vi "GetMethodDependency.vi"(0 "ClassReaderNative in":refnum<class "ClassReaderNative.lvclass">, 1 "Method(s)":variant, 5 "error in (no error)":errorcluster) -> (14 "ClassReaderNative out":refnum<class "ClassReaderNative.lvclass">, 15 "DependencyVIs":T1[](array[typedef]), 19 "error out":errorcluster)   [LabVIEW 2012, in "ClassReaderNative.lvclass"]
uses:
  <resource>/Framework/Providers/Open_GDS/ClassProviders/Provider_LvNativeClass/ClassReaderNative_class/ClassReaderNative.lvclass
  <resource>/Framework/Providers/Open_GDS/ClassProviders/Provider_BaseClassInterface/ClassReader_class/MethodDependencyType.ctl
  <resource>/Framework/Providers/Open_GDS/ClassProviders/Common/ScriptingFunctions/SubVIs/Scripting_ViDependencyType.ctl
  <resource>/Framework/Providers/Open_GDS/ClassProviders/Provider_BaseClassInterface/ClassReader_class/ClassReader.lvclass
  <resource>/Framework/Providers/Open_GDS/ClassProviders/Provider_LvNativeClass/ClassReaderNative_class/ClassReaderNative.lvclass/ClassReaderNative.ctl
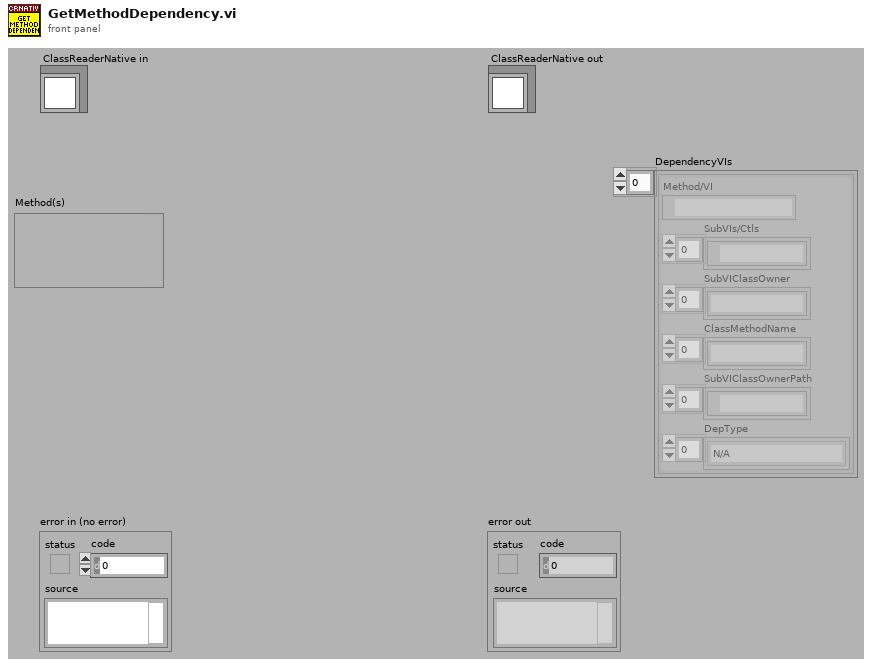
[diagram p1: front panel]
types:
  T1 = typedef "MethodDependencyType.ctl" = cluster{"Method/VI":path, "SubVIs/Ctls":path[], "SubVIClassOwner":string[], "ClassMethodName":string[], "SubVIClassOwnerPath":path[], "DepType":T2[]}
  T2 = typedef "Scripting_ViDependencyType.ctl" = enum16{"N/A", "Launches"}
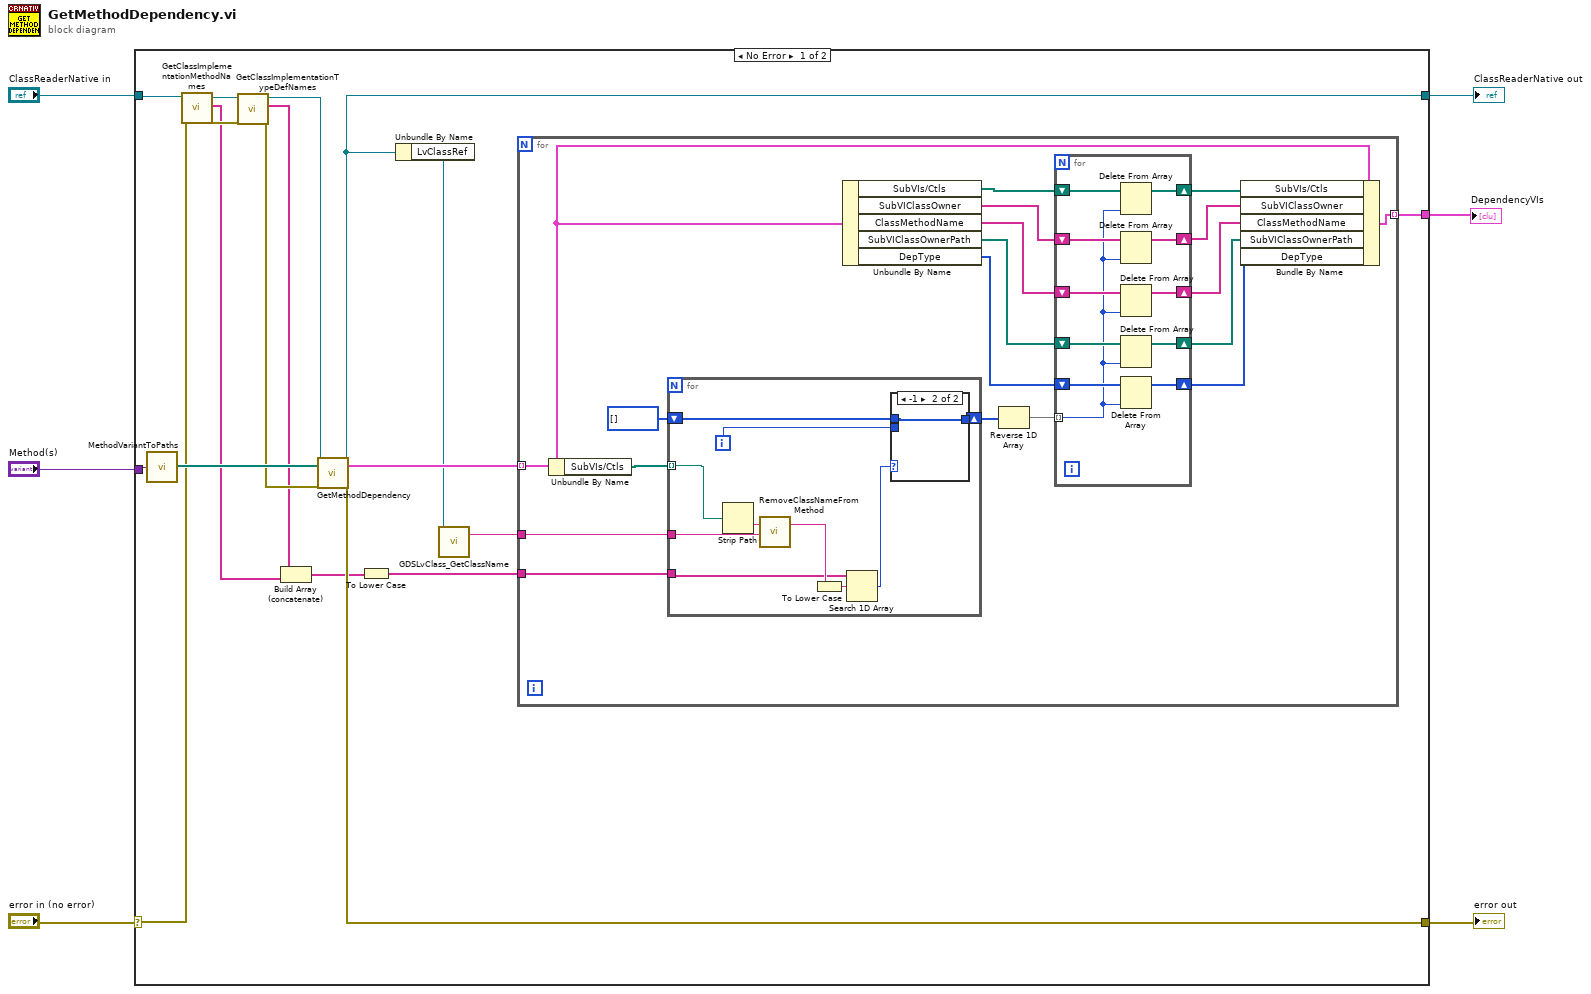
[diagram p0: block diagram]
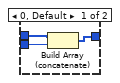
[diagram p2: hidden frame]
diagram:
  n1 = case shown="No Error" "error in (no error)" {
    selector: "error in (no error)" -> [w16 w69]
    tunnel: [w22 w69] -> w5
    tunnel: "ClassReaderNative in" -> [w21 w68]
    tunnel: [w9 w68] -> w3
    tunnel: "Method(s)" -> [w24 _]
    tunnel: [w7 _] -> w1
    frame No Error {
      n2 = call <resource>:"MethodVariantToPaths.vi"("Method(s)"=w24) -> ("Paths"=w23:path[])
      n3 = call-dynamic "GetClassImplementationMethodNames.vi"("error in (no error)"=w16, "ClassReaderNative in"=w21) -> ("error out"=w20:errorcluster, "ImplementationMethodNames"=w12:string[], "ClassReaderNative out"=w19:refnum<class "ClassReaderNative.lvclass">)  [unwired: 7 in]
      n4 = call-dynamic "GetClassImplementationTypeDefNames.vi"("error in (no error)"=w20, "ClassReaderNative in"=w19) -> ("error out"=w17:errorcluster, "ImplementationMethodNames"=w13:string[], "ClassReaderNative out"=w18:refnum<class "ClassReaderNative.lvclass">)  [unwired: 7 in]
      n5 = Build Array (concatenate)(w13, w12) -> (w11:string[])
      n6 = call-parent "GetMethodDependency.vi"("ClassReader in"=w18, "Method(s)"=w23, "error in (no error)"=w17) -> ("ClassReader out"=w9:refnum<class "ClassReaderNative.lvclass">, "DependencyVIs"=w15:T1[], "error out"=w22:errorcluster)  [unwired: 14 in]
      n7 = To Lower Case(string=w11) -> (all lower case string=w10:string[])
      n8 = Unbundle By Name(w9) -> ("LvClassRef"=w14:refnum<vi>)
      n9 = call <resource>:"GDSLvClass_GetClassName.vi"("ViRef/Path,LvClassRef/Path"=w14) -> ("ClassName(without .lvclass)"=w8:string)  [unwired: 16 in, 2 out]
      n10 = for {
        tunnel: w15 -> [w33] mode=indexing
        tunnel: w10 -> [w42]
        tunnel: w8 -> [w41]
        tunnel: [w28] -> w7 mode=indexing
        n11 = Unbundle By Name(w33) -> ("SubVIs/Ctls"=w40:path[])
        n12 = for {
          tunnel: w40 -> [w55] mode=indexing
          shift-right: [w62] -> w38
          shift-left: i32[] [] -> [w63]
          tunnel: w42 -> [w59]
          tunnel: w41 -> [w57]
          i -> [w54]
          n13 = Strip Path(path=w55) -> (name=w58:string)  [unwired: 1 out]
          n14 = call <resource>:"RemoveClassNameFromMethod.vi"("MethodVINameIn"=w58, "ClassName"=w57) -> ("MethodVINameOut"=w61:string)  [unwired: 17 in]
          n15 = To Lower Case(string=w61) -> (all lower case string=w60:string)
          n16 = Search 1D Array(1D array=w59, element=w60) -> (index of element=w56:i32)  [unwired: 1 in]
          n17 = case shown="-1" w56 {
            tunnel: w63 -> [w66 w67]
            tunnel: [w65 w67] -> w62
            tunnel: w54 -> [w64 _]
            frame 0, Default {
              n18 = Build Array (concatenate)(w66, w64) -> (w65:i32[])
            }
            frame -1 {
            }
          }
        }
        n19 = Unbundle By Name(w33) -> ("SubVIs/Ctls"=w37:path[], "SubVIClassOwner"=w36:string[], "ClassMethodName"=w35:string[], "SubVIClassOwnerPath"=w34:path[], "DepType"=w26:T2[])
        n20 = Reverse 1D Array(array=w38) -> (reversed array=w27:i32[])
        n21 = for {
          shift-right: [w52] -> w32
          shift-left: w37 -> [w53]
          shift-right: [w51] -> w31
          shift-left: w36 -> [w50]
          shift-right: [w48] -> w30
          shift-left: w35 -> [w49]
          shift-right: [w47] -> w29
          shift-left: w34 -> [w46]
          tunnel: w27 -> [w43] mode=indexing
          shift-right: [w44] -> w25
          shift-left: w26 -> [w45]
          n22 = Delete From Array(array=w53, index=w43) -> (array with subset deleted=w52:path[])  [unwired: 1 in, 1 out]
          n23 = Delete From Array(array=w50, index=w43) -> (array with subset deleted=w51:string[])  [unwired: 1 in, 1 out]
          n24 = Delete From Array(array=w49, index=w43) -> (array with subset deleted=w48:string[])  [unwired: 1 in, 1 out]
          n25 = Delete From Array(array=w46, index=w43) -> (array with subset deleted=w47:path[])  [unwired: 1 in, 1 out]
          n26 = Delete From Array(array=w45, index=w43) -> (array with subset deleted=w44:T2[])  [unwired: 1 in, 1 out]
        }
        n27 = Bundle By Name(cluster=w33, "SubVIs/Ctls"=w32, "SubVIClassOwner"=w31, "ClassMethodName"=w30, "SubVIClassOwnerPath"=w29, "DepType"=w25) -> (w28:T1)
      }
    }
    frame Error {
    }
  }
  "ClassReaderNative out" <- w3
  "DependencyVIs" <- w1
  "error out" <- w5
